vi "KB-ShowBasePoint2.vi"(8 "error in (no error)":errorcluster, 10 "Create Flatnesss Base Point":cluster{"X":dbl, "Y":dbl, "Z":dbl}[](array[cluster]), 11 "Image In":T1(plugin-control)) -> (0 "error out":errorcluster, 3 "Image Out":T1(plugin-control))   [LabVIEW 2015]
panel:
  out "数值":i32
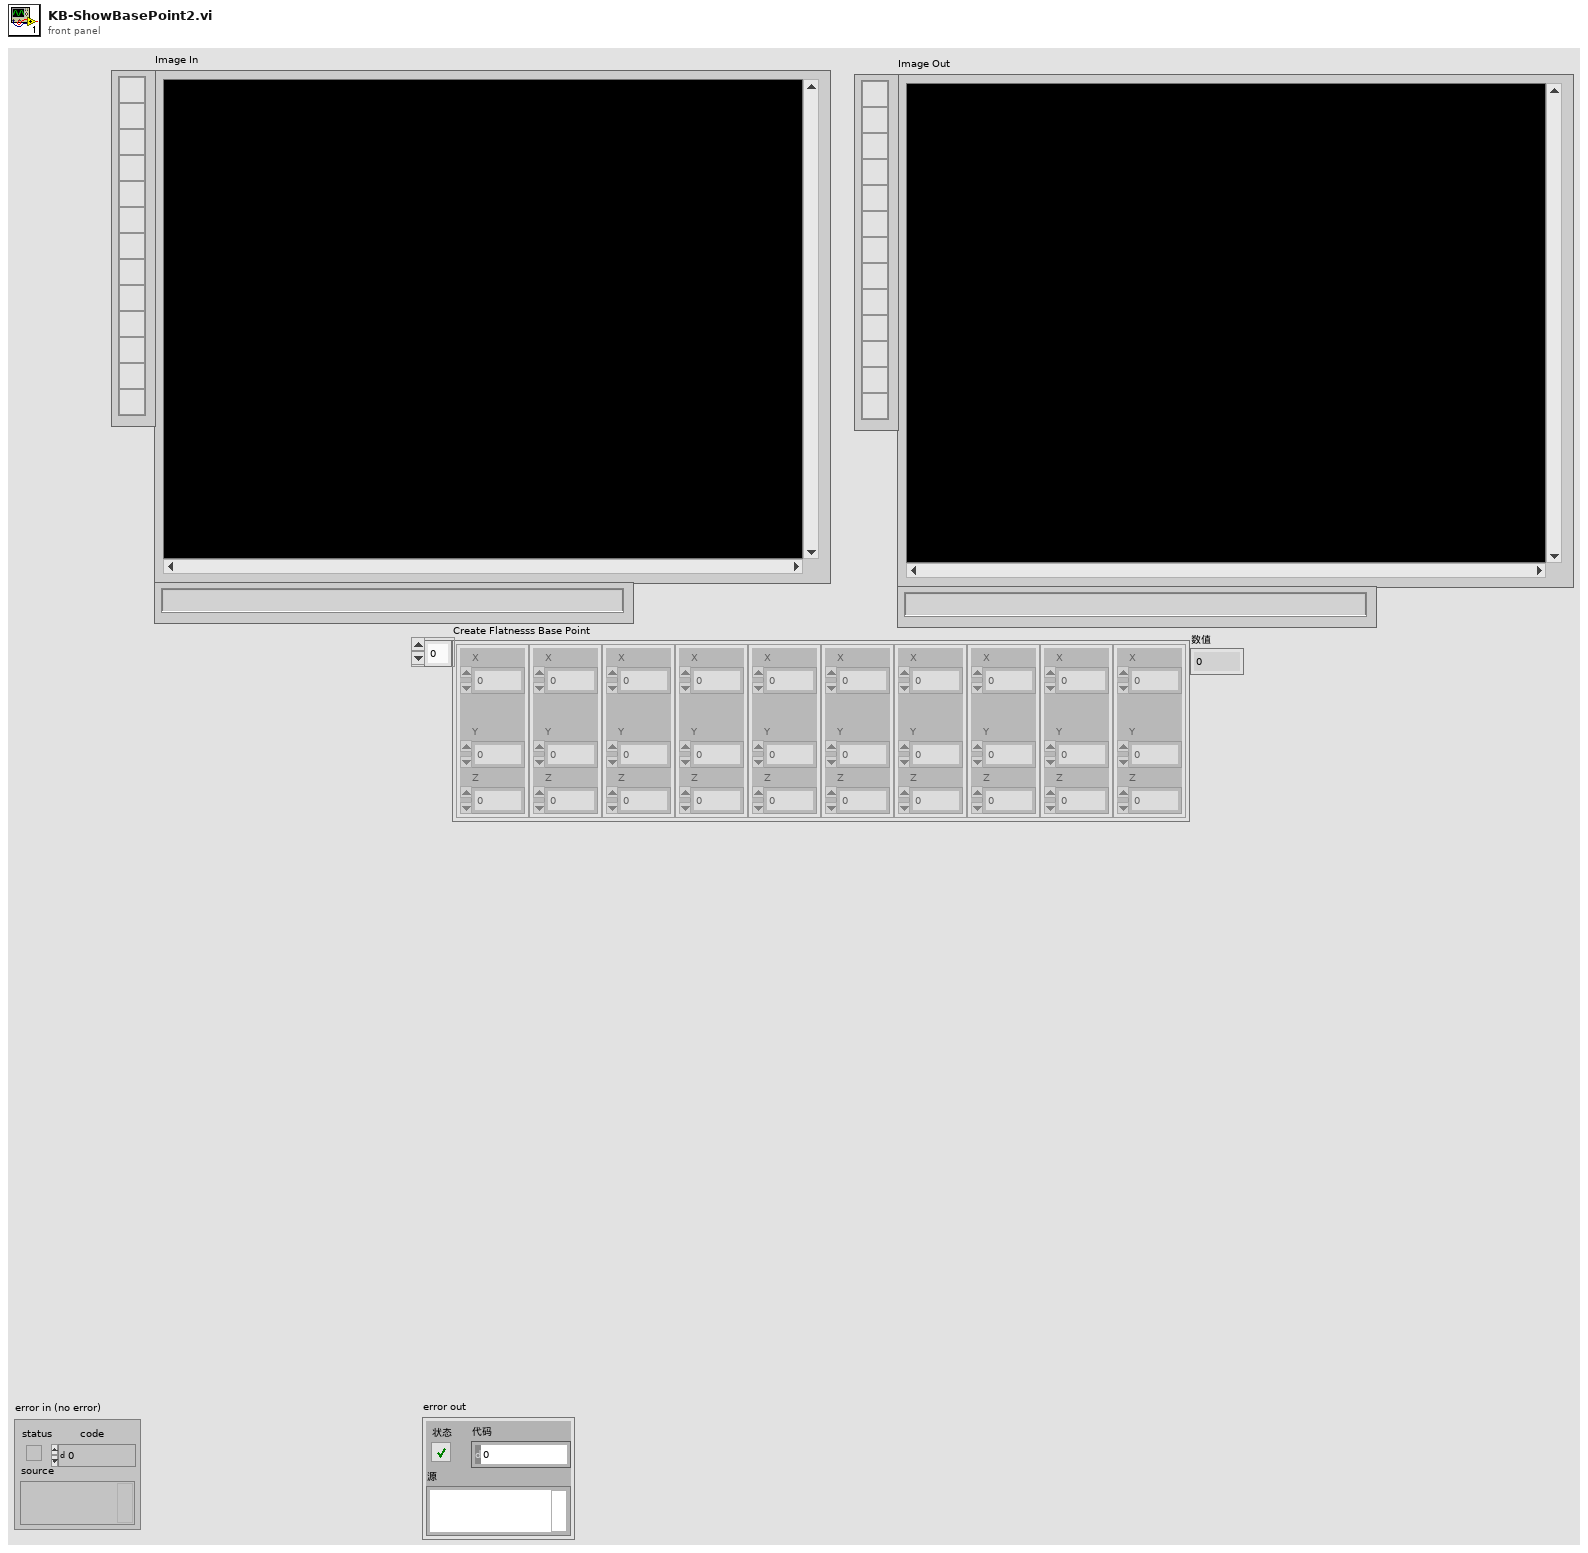
[diagram p1: front panel]
types:
  T1 = typedef "IMAQ Image.ctl" = refnum<image>
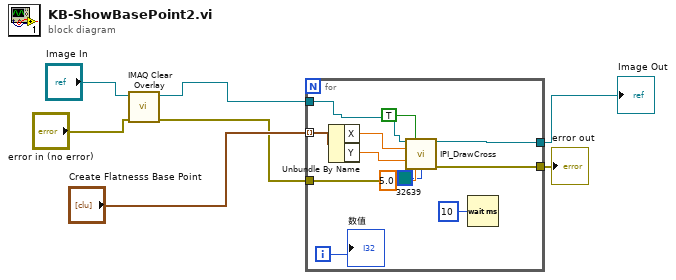
[diagram p0: block diagram]
diagram:
  n1 = call "IMAQ Clear Overlay"("error in (no error)"="error in (no error)", "Image"="Image In") -> ("error out"=w1:errorcluster, "Image Out"=w3:T1)  [unwired: 8 in]
  n2 = for {
    tunnel: "Create Flatnesss Base Point" -> [w19] mode=indexing
    tunnel: [w11] -> w5
    tunnel: w1 -> [w14]
    tunnel: [w13] -> w6
    tunnel: w3 -> [w12]
    i -> [w10]
    n3 = Unbundle By Name(w19) -> ("X"=w18:dbl, "Y"=w17:dbl)
    n4 = call "IPI_DrawCross.vi"("Image In"=w12, "Show Cross"=TRUE, "X"=w18, "Y"=w17, "error in (no error)"=w14, "Radius"=5.0, "颜色盒"=u32 32639) -> ("Image Out"=w11:T1, "error out"=w13:errorcluster)  [unwired: 7 in]
    n5 = Wait (ms)(milliseconds to wait=u32 10 ("等待时间（毫秒）")) -> ()  [unwired: 1 out]
    "数值" <- w10
  }
  "error out" <- w6
  "Image Out" <- w5
